vi "NF87xx.evt call Set Velocity.vi"(0 "i ref in":refnum<vi>, 1 "Instance":string="N/A", 2 "velocity (0 .. 2000)":dbl=10.0 min=10.0 max=2000.0, 3 "Motor (0)":i32, 5 "error in (no error)":errorcluster, 6 "System":string="N/A") -> (14 "i ref out":refnum<vi>, 19 "error out":errorcluster)   [LabVIEW 2014, in "NF87XX.lvlib"]
doc: "This VI sets the \"SetVelocity\" case by a simple call. The instance has to be something else but N/A and the Motor 0, 1 or 2. The parameter are corced to the allowed range."
uses:
  NF87XX.lvlib
  CS_Core/CSSystem/CoreLib/CoreLib.int 2 byte array.vi
  CS_Core/CSSystem/CoreLib/CoreLib.double 2 byte array.vi
  CS_Core/CSSystem/CoreLib/CoreLib.string 2 byte array.vi
  CS_Core/BaseProcess/BaseProcess.lvlib
  CS_Core/CSSystem/CoreLib/CoreLib.lvlib
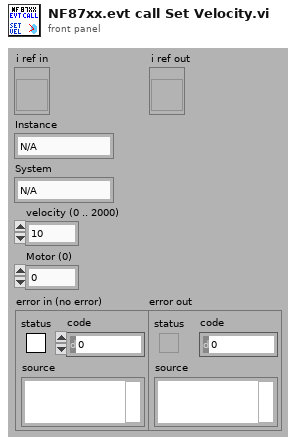
[diagram p1: front panel]
types:
  T1 = enum16{"simple", "synchronous", "asynchronous", "notification"}
  T2 = typedef "CoreDefs.rawDataType.ctl" = i8[]
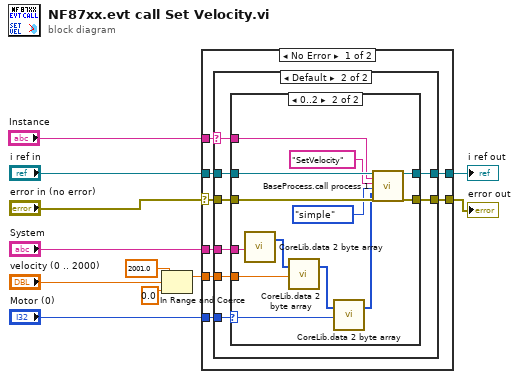
[diagram p0: block diagram]
diagram:
  n1 = In Range and Coerce(upper limit=2001.0, x="velocity (0 .. 2000)", lower limit=0.0) -> (coerced(x)=w3:dbl)  [unwired: 1 out]
  n2 = case shown="No Error" "error in (no error)" {
    selector: "error in (no error)" -> [w13 w45]
    tunnel: [w19 w46] -> w11
    tunnel: [w18 w45] -> w10
    tunnel: "i ref in" -> [w17 w46]
    tunnel: "Motor (0)" -> [w16 _]
    tunnel: w3 -> [w15 _]
    tunnel: "Instance" -> [w14 _]
    tunnel: "System" -> [w12 _]
    frame No Error {
      n3 = case shown="Default" w14 {
        selector: w14 -> [_ w24]
        tunnel: [w21 w29] -> w19
        tunnel: [w20 w28] -> w18
        tunnel: w17 -> [w21 w27]
        tunnel: w13 -> [w20 w26]
        tunnel: w16 -> [_ w23]
        tunnel: w15 -> [_ w25]
        tunnel: w12 -> [_ w22]
        frame "N/A" {
        }
        frame Default {
          n4 = case shown="0..2" w23 {
            selector: w23 -> [_ w38]
            tunnel: [w30 w44] -> w29
            tunnel: [w31 w43] -> w28
            tunnel: w27 -> [w30 w42]
            tunnel: w26 -> [w31 w41]
            tunnel: w25 -> [_ w40]
            tunnel: w24 -> [_ w39]
            tunnel: w22 -> [_ w37]
            frame Default {
            }
            frame 0..2 {
              n5 = call-poly "CoreLib.data 2 byte array.vi"("string"=w37) -> ("byteArray out"=w33:T2)  [unwired: 18 in]
              n6 = call-poly "CoreLib.data 2 byte array.vi"("byteArray"=w33, "f64"=w40) -> ("byteArray out"=w34:T2)  [unwired: 17 in]
              n7 = call-poly "CoreLib.data 2 byte array.vi"("byteArray"=w34, "i32"=w38) -> ("byteArray out"=w32:T2)  [unwired: 17 in]
              n8 = call "BaseProcess.call process 1.vi"("i ref in"=w42, "Object"=w39, "Selector"="SetVelocity", "CallType"=T1."simple", "Data"=w32, "error in (no error)"=w41) -> ("i ref out"=w44:refnum<vi>, "error out"=w43:errorcluster)  [unwired: 11 in, 1 out]
            }
          }
        }
      }
    }
    frame Error {
    }
  }
  "error out" <- w10
  "i ref out" <- w11
